vi "Scale Wave Properties.vi"(0 "f0":sgl, 1 "DCoffset":sgl, 2 "Vspan":sgl, 3 "Mod":T1) -> (5 "FXP Props":T2)   [LabVIEW 2015]
doc: "This VI converts modulation frequencies and voltage signals into something that can be used on the PAS FPGA which uses integer and fxd pt math. For the direct digital synthesis of the waves, the FPGA will use a 32-bit accumulator. The voltage span will be converted to a a number that will scale the I16 FPGA input while the DC offset is converted to I16."
uses:
  Controls/FxdPt Props.ctl
  Reusable/PAS/Main/Controls/Laser Modulation.ctl
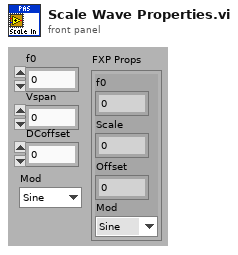
[diagram p1: front panel]
types:
  T1 = typedef "Laser Modulation.ctl" = enum8{"Sine", "Square"}
  T2 = typedef "FxdPt Props.ctl" = cluster{"f0":fxp<+,32,0>, "Scale":fxp<+,14,1>, "Offset":i16, "Mod":T1}
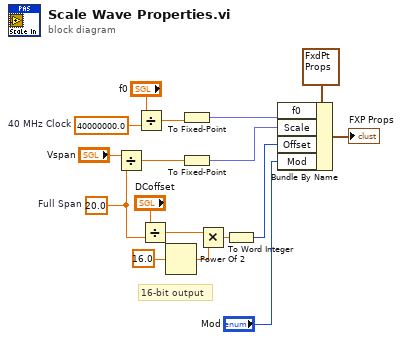
[diagram p0: block diagram]
diagram:
  w2 = sgl 20.0  # Full Span
  w17 = sgl 40000000.0  # 40 MHz Clock
  # "16-bit output"
  n1 = Divide(x="Vspan", y=w2) -> (x/y=w13:sgl)
  n2 = Divide(x="f0", y=w17) -> (x/y=w4:sgl)
  n3 = Divide(x="DCoffset", y=w2) -> (x/y=w8:sgl)
  n4 = Power Of 2(x=sgl 16.0) -> (2^x=w11:sgl)
  n5 = To Fixed-Point(number=w4) -> (fixed-point=w3:fxp<+,32,0>)  [unwired: 1 in]
  n6 = To Fixed-Point(number=w13) -> (fixed-point=w12:fxp<+,14,1>)  [unwired: 1 out]
  n7 = Multiply(x=w8, y=w11) -> (x*y=w10:sgl)
  n8 = To Word Integer(number=w10) -> (16bit integer=w9:i16)
  n9 = Bundle By Name(cluster=T2 {"f0"=0.0, "Scale"=0.0, "Offset"=0, "Mod"=enum."Sine"} ("Scaled Sinewave Props"), "f0"=w3, "Scale"=w12, "Offset"=w9, "Mod"="Mod") -> (→"FXP Props":T2)
